vi "LED Stand Alone.vi"() -> ()   [LabVIEW 2015]
uses:
  <vilib>/myRIO/Instrument Drivers/Onboard IO/DIO/typedefs/DIO Reference.ctl
  <vilib>/myRIO/Common/Instrument Driver Framework/Utilities/typedefs/myRIO Generic Hardware Reference.ctl
  <vilib>/myRIO/Common/Instrument Driver Framework/Utilities/typedefs/Hardware Version Enum.ctl
  <vilib>/myRIO/Common/Instrument Driver Framework/Utilities/typedefs/myRIO v1.0 Reference.ctl
  <vilib>/myRIO/Common/Instrument Driver Framework/Utilities/typedefs/Generic FPGA Reference.ctl
  <vilib>/myRIO/Common/Instrument Driver Framework/myRIO v1.0/DIO/typedefs/DIO Channels List.ctl
  <vilib>/myRIO/Common/Instrument Driver Framework/myRIO v1.0/DIO/typedefs/DIO Channels Enum.ctl
  <vilib>/userdefined/High Color/nirio_resource_hc.ctl
  <vilib>/myRIO/Common/Instrument Driver Framework/myRIO v1.0/DIO/vis/myRIO v1.1 Open DIO.vi
  <vilib>/myRIO/Common/Instrument Driver Framework/myRIO v1.0/DIO/vis/myRIO v1.0 Close DIO.vi
  <vilib>/myRIO/Common/Instrument Driver Framework/Utilities/vis/Validate Channels.vi
  <vilib>/myRIO/Common/Instrument Driver Framework/myRIO v1.0/DIO/vis/myRIO v1.0 Reserve DIO.vi
  <vilib>/myRIO/Common/Instrument Driver Framework/myRIO v1.0/DIO/vis/myRIO v1.0 Unreserve DIO.vi
  <vilib>/myRIO/Common/Instrument Driver Framework/myRIO v1.0/Resource Manager/vis/myRIO v1.0 Reserve Channel List.vi
  <vilib>/myRIO/Common/Instrument Driver Framework/myRIO v1.0/DIO/vis/myRIO v1.0 Build MUX Configuration DIO.vi
  <vilib>/myRIO/Common/Instrument Driver Framework/myRIO v1.0/Resource Manager/vis/myRIO v1.0 Unreserve Channel List.vi
  <vilib>/myRIO/Common/Instrument Driver Framework/myRIO v1.0/Resource Manager/vis/myRIO v1.0 Reserve Channel.vi
  <vilib>/myRIO/Common/Instrument Driver Framework/myRIO v1.0/Resource Manager/vis/myRIO v1.0 Unreserve Channel.vi
  <vilib>/myRIO/Common/Instrument Driver Framework/myRIO v1.0/Resource Manager/vis/myRIO v1.0 Create Configuration List.vi
  <vilib>/myRIO/Common/Instrument Driver Framework/myRIO v1.0/Resource Manager/vis/myRIO v1.0 Build Mutex Name.vi
  <vilib>/Utility/VariantDataType/GetNumericInfo.vi
  <vilib>/Utility/error.llb/Error Cluster From Error Code.vi
  <vilib>/myRIO/Common/Instrument Driver Framework/myRIO v1.0/myRIO v1.1 Open.vi
  <vilib>/myRIO/Common/Instrument Driver Framework/Utilities/vis/IO Manager.vi
  <vilib>/myRIO/Common/Instrument Driver Framework/Utilities/vis/Configuration Manager.vi
  <vilib>/myRIO/Common/Instrument Driver Framework/myRIO v1.0/Resource Manager/vis/myRIO v1.0 Configure IO.vi
  <vilib>/myRIO/Common/Instrument Driver Framework/myRIO v1.0/myRIO v1.0 Close.vi
  <vilib>/myRIO/Common/Instrument Driver Framework/myRIO v1.0/DIO/vis/myRIO v1.0 Read DIO.vi
  <vilib>/myRIO/Common/Instrument Driver Framework/myRIO v1.0/DIO/vis/myRIO v1.0 Write DIO.vi
  <vilib>/myRIO/Common/Instrument Driver Framework/myRIO v1.0/DIO/vis/myRIO v1.0 Shutdown DIO.vi
  <vilib>/myRIO/Instrument Drivers/Onboard IO/DIO/vis/myRIO DIO Open.xnode
  <vilib>/myRIO/Instrument Drivers/Onboard IO/DIO/DIO.lvlib
panel:
  out "Array":bool[](array[boolean])
  out "subarray":bool[](array[boolean])
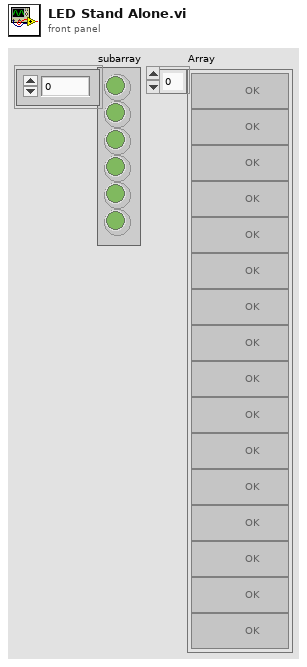
[diagram p1: front panel]
types:
  T1 = typedef "nirio_resource_hc.ctl" = tag
  T2 = typedef "Hardware Version Enum.ctl" = enum16{"Unknown", "myRIO-1900", "myRIO-1950", "roboRIO"}
  T3 = typedef "DIO.lvlib/DIO Reference.ctl" = cluster{"myRIO Reference":T4, "DIO Channels List":T7}
  T4 = typedef "myRIO Generic Hardware Reference.ctl" = cluster{"myRIO Model":T2, "myRIO Hardware Reference":T5}
  T5 = typedef "myRIO v1.0 Reference.ctl" = cluster{"Generic FPGA Reference":T6, "Allow multiple opens":bool}
  T6 = typedef "Generic FPGA Reference.ctl" = refnum<k20>
  T7 = typedef "DIO Channels List.ctl" = T8[]
  T8 = typedef "DIO Channels Enum.ctl" = enum16{"Not Connected", "C/DIO0", "C/DIO1", "C/DIO2", "C/DIO3", "C/DIO4", "C/DIO5", "C/DIO6", "C/DIO7", "A/DIO0", "A/DIO1", "A/DIO2", "A/DIO3", "A/DIO4", "A/DIO5", "A/DIO6", "A/DIO7", "A/DIO8", "A/DIO9", "A/DIO10", "A/DIO11", "A/DIO12", "A/DIO13", "A/DIO14", "A/DIO15", "B/DIO0", "B/DIO1", "B/DIO2", "B/DIO3", "B/DIO4", "B/DIO5", "B/DIO6", "B/DIO7", "B/DIO8", "B/DIO9", "B/DIO10", "B/DIO11", "B/DIO12", "B/DIO13", "B/DIO14", "B/DIO15", "LED0", "LED1", "LED2", "LED3", "Button0", "DIO/DIO0", "DIO/DIO1", "DIO/DIO2", "DIO/DIO3", "DIO/DIO4", "DIO/DIO5", "DIO/DIO6", "DIO/DIO7", "DIO/DIO8", "DIO/DIO9", "SPI/CS0", "SPI/CS1", "SPI/CS2", "SPI/CS3", "LED RADIO (Green)", "LED RADIO (Red)", "LED COMM (Green)", "LED COMM (Red)", "LED MODE (Green)", "LED MODE (Red)"}
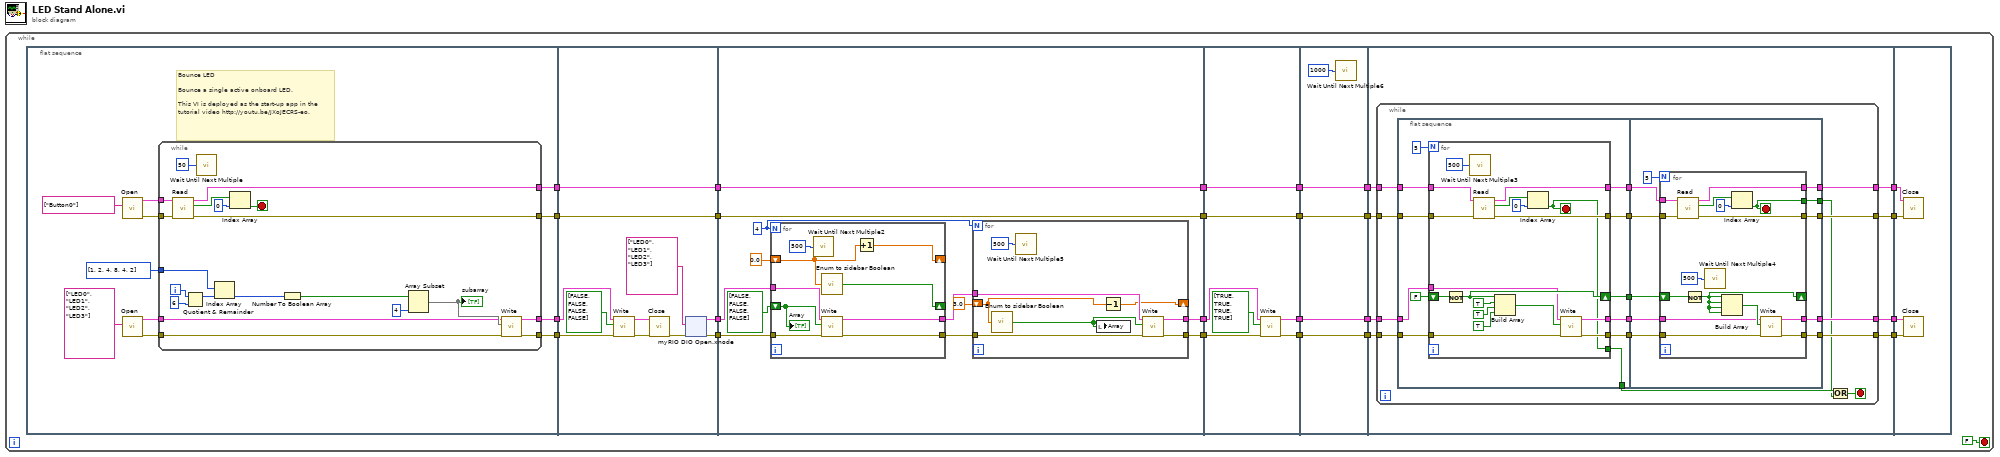
[diagram p0: block diagram]
diagram:
  n1 = while {
    stop <- FALSE stop-if-true
    n2 = flat-sequence {
      tunnel: [w29] -> w8
      tunnel: [w27] -> w7
      tunnel: [w26] -> w6
      tunnel: [w28] -> w4
      tunnel: w8 -> [w64]
      tunnel: w7 -> [w63]
      tunnel: w6 -> [w67]
      tunnel: [w67] -> w5
      tunnel: w4 -> [w66]
      tunnel: [w66] -> w3
      tunnel: [w58] -> w2
      tunnel: [w57] -> w1
      tunnel: [w95] -> w16
      tunnel: [w94] -> w14
      tunnel: w5 -> [w94]
      tunnel: [w90] -> w12
      tunnel: [w89] -> w11
      tunnel: w3 -> [w95]
      tunnel: w2 -> [w92]
      tunnel: w1 -> [w91]
      tunnel: w16 -> [w119]
      tunnel: [w119] -> w15
      tunnel: w14 -> [w118]
      tunnel: [w118] -> w13
      tunnel: w12 -> [w117]
      tunnel: w11 -> [w116]
      tunnel: [w115] -> w10
      tunnel: [w114] -> w9
      tunnel: w15 -> [w124]
      tunnel: [w124] -> w20
      tunnel: w13 -> [w123]
      tunnel: [w123] -> w19
      tunnel: [w122] -> w18
      tunnel: w10 -> [w121]
      tunnel: [w121] -> w17
      tunnel: w9 -> [w122]
      tunnel: w20 -> [w130]
      tunnel: w19 -> [w129]
      tunnel: [w128] -> w25
      tunnel: [w127] -> w24
      tunnel: [w126] -> w23
      tunnel: [w125] -> w22
      tunnel: w18 -> [w131]
      tunnel: w17 -> [w132]
      tunnel: w25 -> [w208]
      tunnel: w24 -> [w207]
      tunnel: w23 -> [w206]
      tunnel: w22 -> [w205]
      frame #0 {
        # "Bounce LED\n\nBounce a single active onboard LED.\n\nThis VI is deployed as the start-up app in the\ntutorial video http://youtu.be/JXoJECRS-eo."
        n3 = call <vilib>:"Open.vi"("Channel Names"=tag[] ["Button0"]) -> ("error out"=w30:errorcluster, "DIO Ref Out"=w31:T3)  [unwired: 9 in]
        n4 = call <vilib>:"Open.vi"("Channel Names"=tag[] ["LED0", "LED1", "LED2", "LED3"]) -> ("error out"=w33:errorcluster, "DIO Ref Out"=w34:T3)  [unwired: 9 in]
        n5 = while {
          tunnel: w33 -> [w56]
          tunnel: [w45] -> w29
          tunnel: [w44] -> w27
          tunnel: u8[] [1, 2, 4, 8, 4, 2] -> [w48]
          tunnel: w34 -> [w47]
          tunnel: w31 -> [w40]
          tunnel: w30 -> [w39]
          tunnel: [w38] -> w28
          tunnel: [w37] -> w26
          i -> [w55]
          stop <- w41 stop-if-true
          n6 = call <vilib>:"Read.vi"("error in (no error)"=w39, "DIO Ref In"=w40) -> ("error out"=w37:errorcluster, "Values"=w43:bool[], "DIO Ref Out"=w38:T3)  [unwired: 7 in]
          n7 = Quotient & Remainder(x=w55, y=6) -> (x-y*floor(x/y)=w53:i32)  [unwired: 1 out]
          n8 = call "Wait Until Next Multiple"("Count(mSec)"=u32 50) -> ()  [unwired: 1 out]
          n9 = Index Array "Index Array"(array=w48, index=w53) -> (element=w52:u8)
          n10 = Index Array(array=w43, index=0) -> (element=w41:bool)
          n11 = Number To Boolean Array(number=w52) -> (Boolean array=w51:bool[])
          n12 = Array Subset "Array Subset"(array=w51, length=4) -> (w49:bool[])  [unwired: 1 in]
          "subarray" <- w49
          n13 = call <vilib>:"Write.vi"("error in (no error)"=w56, "Values"=w49, "DIO Ref In"=w47) -> ("error out"=w44:errorcluster, "DIO Ref Out"=w45:T3)  [unwired: 6 in]
        }
      }
      frame #1 {
        n14 = call <vilib>:"Write.vi"("error in (no error)"=w63, "Values"=bool[] [FALSE, FALSE, FALSE, FALSE], "DIO Ref In"=w64) -> ("error out"=w62:errorcluster, "DIO Ref Out"=w61:T3)  [unwired: 6 in]
        n15 = call <vilib>:"Close.vi"("error in (no error)"=w62, "DIO Ref In"=w61) -> ("error out"=w60:errorcluster)  [unwired: 9 in]
        n16 = xnode "myRIO DIO Open.xnode"("error in (no error)"=w60, "Channel Names"=tag[] ["LED0", "LED1", "LED2", "LED3"]) -> ("error out"=w57:errorcluster, "DIO Ref Out"=w58:T3)  [unwired: 1 in]
      }
      frame #2 {
        w86 = 4
        n17 = for {
          N: w86 -> [_]
          shift-right: [w108] -> _
          shift-left: 0.0 -> [w106]
          tunnel: w92 -> [w112]
          tunnel: w91 -> [w111]
          tunnel: [w110] -> w88
          tunnel: [w109] -> w87
          shift-right: [w105] -> _
          shift-left: bool[] [FALSE, FALSE, FALSE, FALSE] ("Array") -> [w104]
          n18 = call "Wait Until Next Multiple2"("Count(mSec)"=u32 500) -> ()  [unwired: 1 out]
          n19 = call "Enum to sidebar Boolean.vi"("Button No (T)"=w106) -> ("Array"=w105:bool[])
          n20 = call <vilib>:"Write.vi"("error in (no error)"=w111, "Values"=w104, "DIO Ref In"=w112) -> ("error out"=w109:errorcluster, "DIO Ref Out"=w110:T3)  [unwired: 6 in]
          n21 = Increment(x=w106) -> (x+1=w108:dbl)
          "Array" <- w104
        }
        n22 = for {
          N: w86 -> [_]
          shift-right: [w99] -> _
          shift-left: 3.0 -> [w98]
          tunnel: w88 -> [w103]
          tunnel: w87 -> [w102]
          tunnel: [w101] -> w89
          tunnel: [w100] -> w90
          n23 = call "Enum to sidebar Boolean.vi"("Button No (T)"=w98) -> ("Array"=w96:bool[])
          n24 = call "Wait Until Next Multiple5"("Count(mSec)"=u32 500) -> ()  [unwired: 1 out]
          n25 = local write "Array"(w96) -> ()
          n26 = Decrement(x=w98) -> (x-1=w99:dbl)
          n27 = call <vilib>:"Write.vi"("error in (no error)"=w102, "Values"=w96, "DIO Ref In"=w103) -> ("error out"=w100:errorcluster, "DIO Ref Out"=w101:T3)  [unwired: 6 in]
        }
      }
      frame #3 {
        n28 = call <vilib>:"Write.vi"("error in (no error)"=w117, "Values"=bool[] [TRUE, TRUE, TRUE, TRUE], "DIO Ref In"=w116) -> ("error out"=w114:errorcluster, "DIO Ref Out"=w115:T3)  [unwired: 6 in]
      }
      frame #4 {
        n29 = call "Wait Until Next Multiple6"("Count(mSec)"=u32 1000) -> ()  [unwired: 1 out]
      }
      frame #5 {
        n30 = while {
          tunnel: w132 -> [w145]
          tunnel: w131 -> [w144]
          tunnel: w130 -> [w143]
          tunnel: w129 -> [w142]
          tunnel: [w139] -> w128
          tunnel: [w138] -> w127
          tunnel: [w137] -> w126
          tunnel: [w136] -> w125
          stop <- w133 stop-if-true
          n31 = flat-sequence {
            tunnel: w145 -> [w159]
            tunnel: w144 -> [w158]
            tunnel: [w157] -> w148
            tunnel: [w156] -> w147
            tunnel: [w155] -> w146
            tunnel: w143 -> [w154]
            tunnel: w142 -> [w153]
            tunnel: [w152] -> w141
            tunnel: [w151] -> w140
            tunnel: [w149] -> w135
            tunnel: w148 -> [w189]
            tunnel: w147 -> [w188]
            tunnel: w146 -> [w187]
            tunnel: w141 -> [w186]
            tunnel: w140 -> [w185]
            tunnel: [w184] -> w139
            tunnel: [w183] -> w138
            tunnel: [w182] -> w137
            tunnel: [w181] -> w136
            tunnel: [w179] -> w134
            frame #0 {
              n32 = for {
                N: 5 -> [_]
                shift-right: [w173] -> w155
                shift-left: FALSE -> [w174]
                tunnel: w159 -> [w171]
                tunnel: w158 -> [w170]
                tunnel: [w169] -> w157
                tunnel: [w168] -> w156
                tunnel: w154 -> [w165]
                tunnel: w153 -> [w164]
                tunnel: [w163] -> w152
                tunnel: [w162] -> w151
                tunnel: [w161] -> w149
                stop <- w161 stop-if-true
                n33 = Not(x=w174) -> (.not. x?=w173:bool)
                n34 = call "Wait Until Next Multiple3"("Count(mSec)"=u32 500) -> ()  [unwired: 1 out]
                n35 = call <vilib>:"Read.vi"("error in (no error)"=w164, "DIO Ref In"=w165) -> ("error out"=w162:errorcluster, "Values"=w166:bool[], "DIO Ref Out"=w163:T3)  [unwired: 7 in]
                n36 = Build Array(w173, TRUE, TRUE, TRUE) -> (w178:bool[])
                n37 = Index Array(array=w166, index=0) -> (element=w161:bool)
                n38 = call <vilib>:"Write.vi"("error in (no error)"=w170, "Values"=w178, "DIO Ref In"=w171) -> ("error out"=w168:errorcluster, "DIO Ref Out"=w169:T3)  [unwired: 6 in]
              }
            }
            frame #1 {
              n39 = for {
                N: 5 -> [_]
                shift-right: [w199] -> _
                shift-left: w187 -> [w203]
                tunnel: w189 -> [w201]
                tunnel: w188 -> [w200]
                tunnel: w186 -> [w196]
                tunnel: w185 -> [w195]
                tunnel: [w194] -> w184
                tunnel: [w193] -> w183
                tunnel: [w192] -> w182
                tunnel: [w191] -> w181
                tunnel: [w190] -> w179
                stop <- w190 stop-if-true
                n40 = call <vilib>:"Read.vi"("error in (no error)"=w195, "DIO Ref In"=w196) -> ("error out"=w193:errorcluster, "Values"=w198:bool[], "DIO Ref Out"=w194:T3)  [unwired: 7 in]
                n41 = Not(x=w203) -> (.not. x?=w199:bool)
                n42 = call "Wait Until Next Multiple4"("Count(mSec)"=u32 500) -> ()  [unwired: 1 out]
                n43 = Build Array(w199, w199, w199, w199) -> (w204:bool[])
                n44 = Index Array(array=w198, index=0) -> (element=w190:bool)
                n45 = call <vilib>:"Write.vi"("error in (no error)"=w200, "Values"=w204, "DIO Ref In"=w201) -> ("error out"=w191:errorcluster, "DIO Ref Out"=w192:T3)  [unwired: 6 in]
              }
            }
          }
          n46 = Or(x=w135, y=w134) -> (x .or. y?=w133:bool)
        }
      }
      frame #6 {
        n47 = call <vilib>:"Close.vi"("error in (no error)"=w207, "DIO Ref In"=w208) -> ()  [unwired: 9 in, 1 out]
        n48 = call <vilib>:"Close.vi"("error in (no error)"=w205, "DIO Ref In"=w206) -> ()  [unwired: 9 in, 1 out]
      }
    }
  }
